vi "LSX Get Serial Nr.vi"(8 "error in (no error)":errorcluster, 9 "lMaxLen":i32, 10 "pcSerialNr":string, 11 "lLSID":i32) -> (0 "error out":errorcluster, 2 "pcSerialNr out":string, 3 "function return":i32)   [LabVIEW 2018, in "Tango.lvlib"]
doc: "TANGOAPI int TANGOCALL LSX_GetSerialNr (int lLSID, char *pcSerialNr, int lMaxLen);"
uses:
  Tango.lvlib
  SubVIs/Tango_DLL.dll
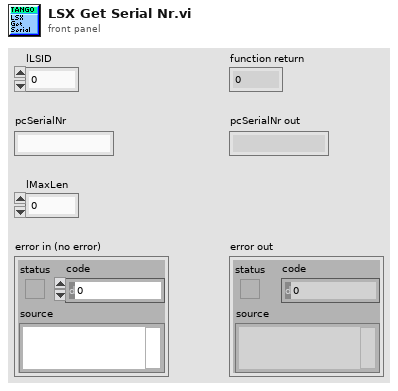
[diagram p1: front panel]
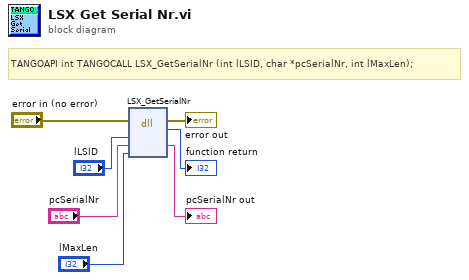
[diagram p0: block diagram]
diagram:
  # "TANGOAPI int TANGOCALL LSX_GetSerialNr (int lLSID, char *pcSerialNr, int lMaxLen);"
  n1 = dll-call lib="C:/Users/Familie/Documents/LabviewIX81/lib/TANGO Stage/SubVIs/Tango_DLL.*" fn="LSX_GetSerialNr"(error in="error in (no error)", "lLSID"="lLSID", "pcSerialNr"="pcSerialNr", "lMaxLen"="lMaxLen") -> (error out=→"error out":errorcluster, →"function return":i32, "pcSerialNr"=→"pcSerialNr out":string)  [unwired: 4 in, 1 out]
